vi "Play Sound Effx.vi"(7 "event":enum16{"Play", "Stop"}(ring), 8 "error in (no error)":errorcluster, 9 "path":path, 10 "Sound Effect Off":T1, 11 "Sounds In":T2[](array[typedef]) {"Task ID" format="%.0x"}) -> (0 "error out":errorcluster, 3 "Sounds Out":T2[](array[typedef]) {"Task ID" format="%.0x"})   [LabVIEW 2021, in "Sound Manager.lvlib"]
uses:
  Sound Manager.lvlib
  Typedefs/Sound Data.ctl
  Typedefs/Sound Effects.ctl
  <vilib>/sound2/lvsound2.llb/Sound Output Task ID.ctl
  <vilib>/sound2/lvsound2.llb/Sound Output Set Volume (Single).vi
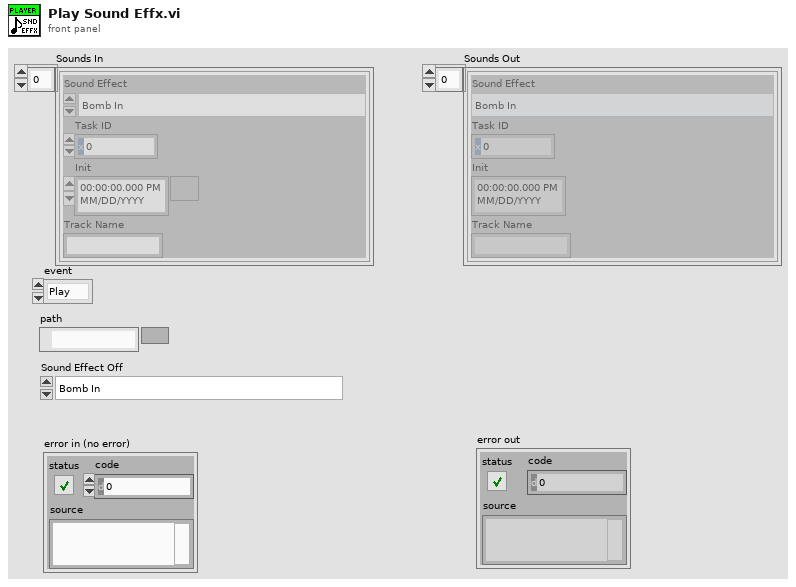
[diagram p1: front panel]
types:
  T1 = typedef "Sound Manager.lvlib/Sound Effects.ctl" = enum16{"Bomb In", "Bomb Out", "Bomb Touched", "Game Over", "Victory", "Eat", "10 Fruits", "Eat2", "Eat3", "Eat4", "MaxShield", "Shield", "10p", "Grape In", "Grape Out", "20p", "30p", "40p", "50p", "60p", "70p", "80p", "90p", "100p", "All shields cracked", "Mouse In", "Mouse Out", "Mouse Eaten", "Grape Eaten", "States Recover", "Broken Shield", "Bonus", "Happy Time", "explode", "Game over musica", "Back Music", "Shield Catch", "Evil lough", "Cricket In", "Cricket eaten", "Lets Go", "Jump1", "Jump2", "Jump3", "Unstoppable", "Troll Music", "winner"}
  T2 = typedef "Sound Manager.lvlib/Sound Data.ctl" = cluster{"Sound Effect":T1, "Task ID":T3, "Init":timestamp, "Track Name":string}
  T3 = typedef "Sound Output Task ID.ctl" = u32
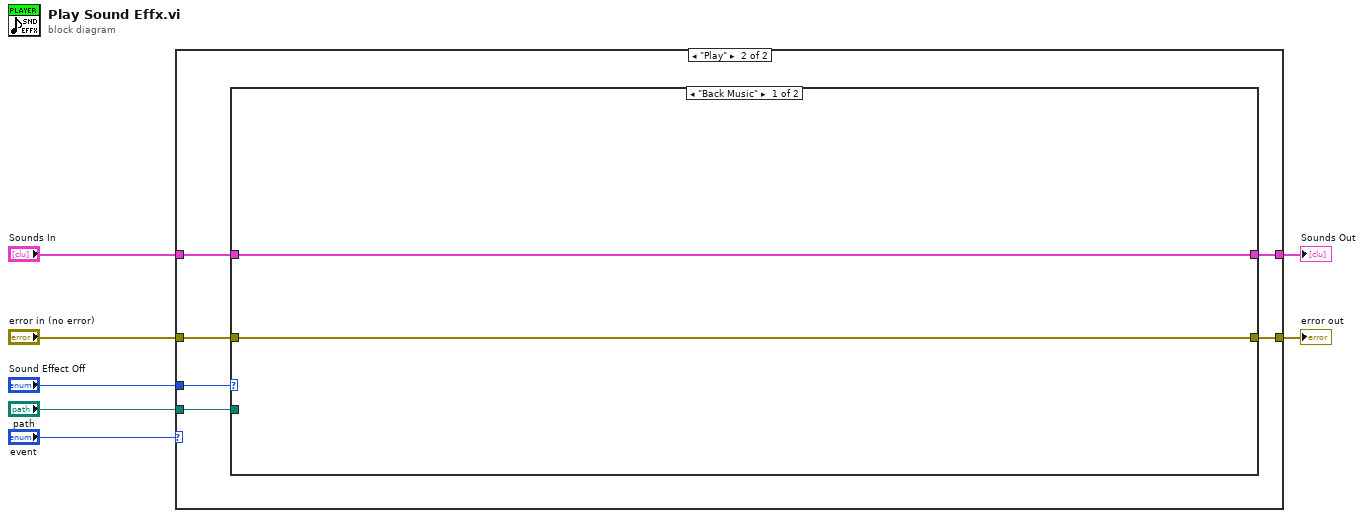
[diagram p0: block diagram]
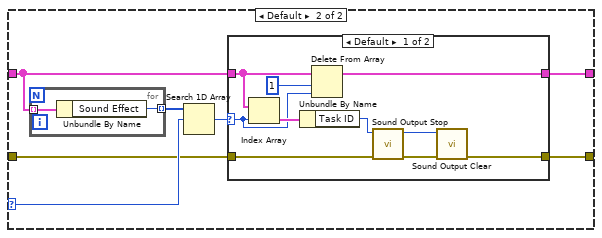
[diagram p3: hidden frame]
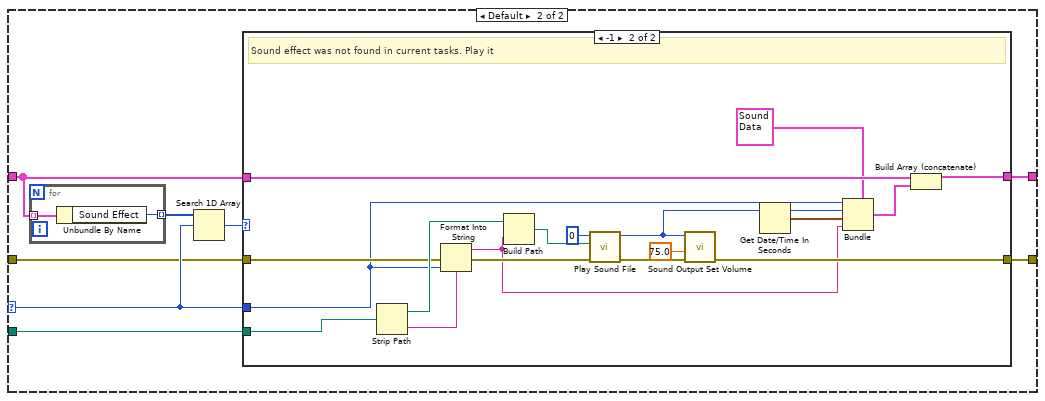
[diagram p5: hidden frame]
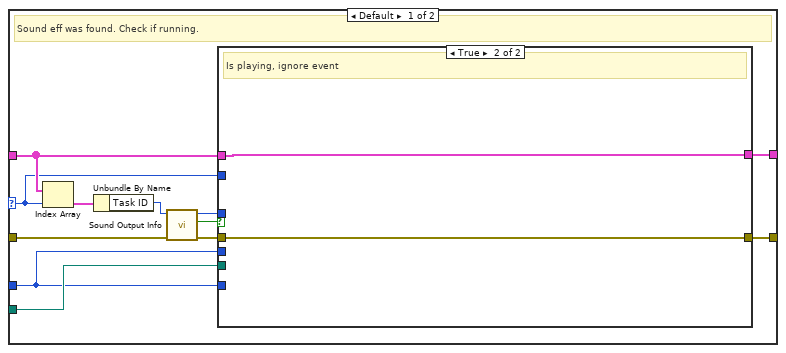
[diagram p6: hidden frame]
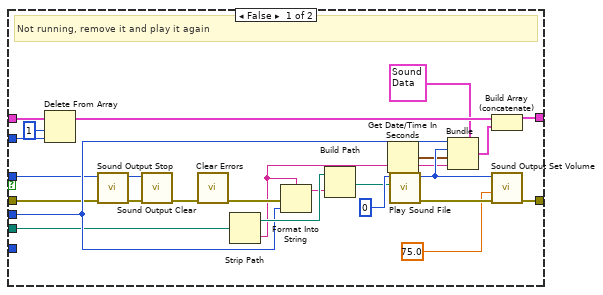
[diagram p7: hidden frame]
diagram:
  n1 = case shown="\"Play\"" "event" {
    tunnel: [w12 w41] -> w7
    tunnel: "Sounds In" -> [w11 w40]
    tunnel: "Sound Effect Off" -> [w10 w39]
    tunnel: "path" -> [_ w38]
    tunnel: [w8 w37] -> w1
    tunnel: "error in (no error)" -> [w9 w36]
    frame "Stop" {
      n2 = case shown="\"Back Music\"" w10 {
        selector: w10 -> [_ w21]
        tunnel: w11 -> [w14 w18]
        tunnel: [w14 w17] -> w12
        tunnel: w9 -> [w13 w16]
        tunnel: [w13 w15] -> w8
        frame "Back Music" {
        }
        frame Default {
          n3 = for {
            tunnel: w18 -> [w35] mode=indexing
            tunnel: [w34] -> w20 mode=indexing
            n4 = Unbundle By Name(w35) -> ("Sound Effect"=w34:T1)
          }
          n5 = Search 1D Array(1D array=w20, element=w21) -> (index of element=w19:i32)  [unwired: 1 in]
          n6 = case shown="Default" w19 {
            selector: w19 -> [w25 _]
            tunnel: w18 -> [w27 w33]
            tunnel: [w24 w33] -> w17
            tunnel: w16 -> [w23 w32]
            tunnel: [w22 w32] -> w15
            frame Default {
              n7 = Index Array(array=w27, index=w25) -> (element=w31:T2)
              n8 = Unbundle By Name(w31) -> ("Task ID"=w30:T3)
              n9 = Delete From Array(array=w27, length=1, index=w25) -> (array with subset deleted=w24:T2[])  [unwired: 1 out]
              n10 = call <vilib>:"Sound Output Stop.vi"("error in (no error)"=w23, "task ID"=w30) -> ("error out"=w28:errorcluster, "task ID out"=w29:T3)  [unwired: 8 in]
              n11 = call <vilib>:"Sound Output Clear.vi"("error in (no error)"=w28, "task ID"=w29) -> ("error out"=w22:errorcluster)  [unwired: 9 in]
            }
            frame -1 {
            }
          }
        }
      }
    }
    frame "Play" {
      n12 = case shown="\"Back Music\"" w39 {
        selector: w39 -> [_ w47]
        tunnel: w40 -> [w43 w49]
        tunnel: [w43 w48] -> w41
        tunnel: w38 -> [_ w46]
        tunnel: [w42 w45] -> w37
        tunnel: w36 -> [w42 w44]
        frame "Back Music" {
        }
        frame Default {
          n13 = for {
            tunnel: w49 -> [w110] mode=indexing
            tunnel: [w109] -> w51 mode=indexing
            n14 = Unbundle By Name(w110) -> ("Sound Effect"=w109:T1)
          }
          n15 = Search 1D Array(1D array=w51, element=w47) -> (index of element=w50:i32)  [unwired: 1 in]
          n16 = case shown="-1" w50 {
            selector: w50 -> [w52 _]
            tunnel: w49 -> [w60 w101]
            tunnel: [w59 w100] -> w48
            tunnel: w47 -> [w53 w95]
            tunnel: w46 -> [w56 w99]
            tunnel: [w55 w98] -> w45
            tunnel: w44 -> [w54 w97]
            frame Default {
              # "Sound eff was found. Check if running."
              n17 = Index Array(array=w60, index=w52) -> (element=w63:T2)
              n18 = Unbundle By Name(w63) -> ("Task ID"=w62:T3)
              n19 = call <vilib>:"Sound Output Info.vi"("error in (no error)"=w54, "task ID"=w62) -> ("error out"=w57:errorcluster, "is playing?"=w61:bool, "task ID out"=w58:T3)  [unwired: 6 in, 1 out]
              n20 = case shown="True" w61 {
                tunnel: w60 -> [w82 w90]
                tunnel: [w81 w90] -> w59
                tunnel: w58 -> [w75 _]
                tunnel: w57 -> [w74 w89]
                tunnel: w53 -> [w79 _]
                tunnel: w56 -> [w78 _]
                tunnel: [w72 w89] -> w55
                tunnel: w53 -> [_ _]
                tunnel: w52 -> [w67 _]
                frame False {
                  # "Not running, remove it and play it again"
                  n21 = Delete From Array(array=w82, length=1, index=w67) -> (array with subset deleted=w68:T2[])  [unwired: 1 out]
                  n22 = call <vilib>:"Sound Output Stop.vi"("error in (no error)"=w74, "task ID"=w75) -> ("error out"=w76:errorcluster, "task ID out"=w77:T3)  [unwired: 8 in]
                  n23 = call <vilib>:"Sound Output Clear.vi"("error in (no error)"=w76, "task ID"=w77) -> ("error out"=w73:errorcluster)  [unwired: 9 in]
                  n24 = call <vilib>:"Clear Errors.vi"("error in (no error)"=w73) -> ("error out"=w71:errorcluster)  [unwired: 5 in, 1 out]
                  n25 = Strip Path(path=w78) -> (stripped path=w86:path, name=w64:string)
                  n26 = Format Into String(format string=w64, error in=w71, w79) -> (resulting string=w85:string)  [unwired: 1 in, 1 out]
                  n27 = Build Path(base path=w86, name or relative path=w85) -> (appended path=w84:path)
                  n28 = Get Date/Time In Seconds() -> (seconds since 1Jan1904=w69:timestamp)
                  n29 = call <vilib>:"Play Sound File.vi"("path"=w84, "device ID"=u32 0) -> ("error out"=w87:errorcluster, "task ID"=w83:T3)  [unwired: 8 in]
                  n30 = Bundle(cluster=T2 {"Sound Effect"=enum."Bomb In", "Task ID"=0, "Init"=timestamp(0 s since 1904-01-01), "Track Name"=""} ("Cluster"), "Sound Effect"=w79, "Task ID"=w83, "Init"=w69, "Track Name"=w64) -> (w80:T2)
                  n31 = Build Array (concatenate)(w68, w80) -> (w81:T2[])
                  n32 = call-poly <vilib>:"Sound Output Set Volume.vi"("error in (no error)"=w87, "volume"=75.0, "task ID"=w83) -> ("error out"=w72:errorcluster)  [unwired: 7 in, 1 out]
                }
                frame True {
                  # "Is playing, ignore event"
                }
              }
            }
            frame -1 {
              # "Sound effect was not found in current tasks. Play it"
              n33 = Strip Path(path=w99) -> (stripped path=w104:path, name=w105:string)
              n34 = Format Into String(format string=w105, error in=w97, w95) -> (resulting string=w91:string, error out=w96:errorcluster)  [unwired: 1 in]
              n35 = Build Path(base path=w104, name or relative path=w91) -> (appended path=w94:path)
              n36 = call <vilib>:"Play Sound File.vi"("error in (no error)"=w96, "path"=w94, "device ID"=u32 0) -> ("error out"=w107:errorcluster, "task ID"=w103:T3)  [unwired: 7 in]
              n37 = call-poly <vilib>:"Sound Output Set Volume.vi"("error in (no error)"=w107, "volume"=75.0, "task ID"=w103) -> ("error out"=w98:errorcluster)  [unwired: 7 in, 1 out]
              n38 = Get Date/Time In Seconds() -> (seconds since 1Jan1904=w93:timestamp)
              n39 = Bundle(cluster=T2 {"Sound Effect"=enum."Bomb In", "Task ID"=0, "Init"=timestamp(0 s since 1904-01-01), "Track Name"=""} ("Cluster"), "Sound Effect"=w95, "Task ID"=w103, "Init"=w93, "Track Name"=w91) -> (w102:T2)
              n40 = Build Array (concatenate)(w101, w102) -> (w100:T2[])
            }
          }
        }
      }
    }
  }
  "Sounds Out" <- w7
  "error out" <- w1
